vi "parse -- get list of matches.vi"(10 "regexp":string="(c\\d\\d)\\,?\\s*", 11 "string":string="c11, c22, c33, c23, c13, c12, c44, c55,  c66") -> (0 "Array":string[](array[string])=["c11", "c22", "c33", "c23", "c13", "c12", "c44", "c55", "c66"], 1 "number of free elastic constants":i32=9, 2 "after match":string)   [LabVIEW 2015]
uses:
  <vilib>/regexp/Match Regular Expression.xnode
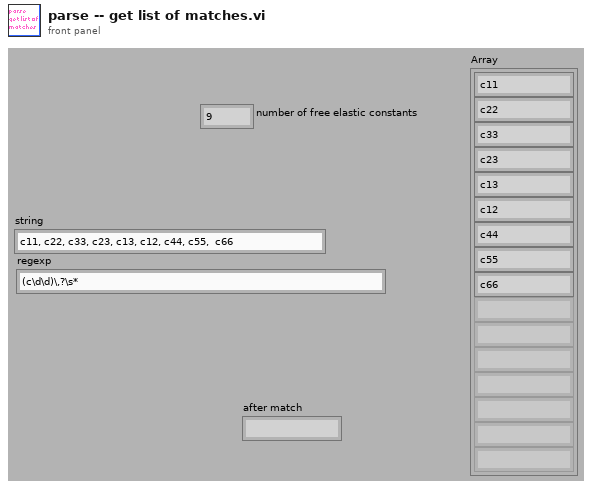
[diagram p1: front panel]
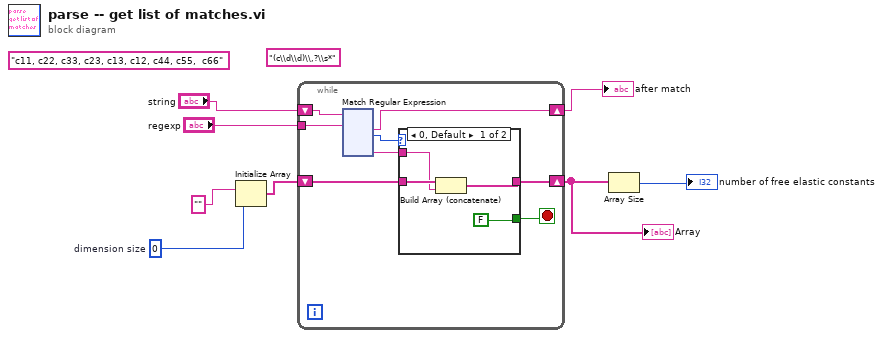
[diagram p0: block diagram]
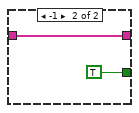
[diagram p2: hidden frame]
diagram:
  w2 = 0  # dimension size
  (unwired) "c11, c22, c33, c23, c13, c12, c44, c55,  c66" ("format string")
  (unwired) "(c\\d\\d)\\,?\\s*" ("format string")
  n1 = Initialize Array("" ("format string"), w2) -> (w1:string[])
  n2 = while {
    tunnel: "regexp" -> [w16]
    shift-right: [w15] -> w6
    shift-left: "string" -> [w14]
    shift-right: [w11] -> w8
    shift-left: w1 -> [w10]
    stop <- w12 stop-if-true
    n3 = xnode "Match Regular Expression"("input string"=w14, "regular expression"=w16) -> ("after match"=w15:string, "offset past match"=w13:i32, "submatch 1"=w9:string)  [unwired: 4 in, 3 out]
    n4 = case shown="0, Default" w13 {
      tunnel: [FALSE TRUE] -> w12
      tunnel: [w17 w21] -> w11
      tunnel: w10 -> [w19 w21]
      tunnel: w9 -> [w18 _]
      frame 0, Default {
        n5 = Build Array (concatenate)(w19, w18) -> (w17:string[])
      }
      frame -1 {
      }
    }
  }
  "after match" <- w6
  "Array" <- w8
  n6 = Array Size(array=w8) -> (size(s)=→"number of free elastic constants":i32)
